vi "Test Command RPIN Response.vi"(8 "error in (no error)":errorcluster, 11 "TestCase in":refnum<class "Test ADC Command.lvclass">) -> (0 "error out":errorcluster, 3 "TestCase out":refnum<class "Test ADC Command.lvclass">)   [LabVIEW 2019, in "Test ADC Command.lvclass"]
uses:
  Test ADC Command.lvclass
  SIMULATED/SIMULATED.lvclass
  <vilib>/addons/_JKI Toolkits/VI Tester/TestCase.llb/TestCase.lvclass
  Serial Devices.lvclass
  C:/Program Files (x86)/National Instruments/LabVIEW 2019/vi.lib/addons/_JKI Toolkits/VI Tester/TestCase.llb/TestCase.lvclass
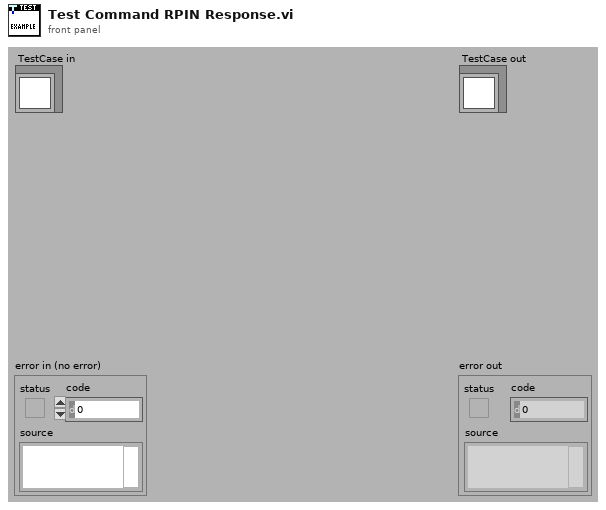
[diagram p1: front panel]
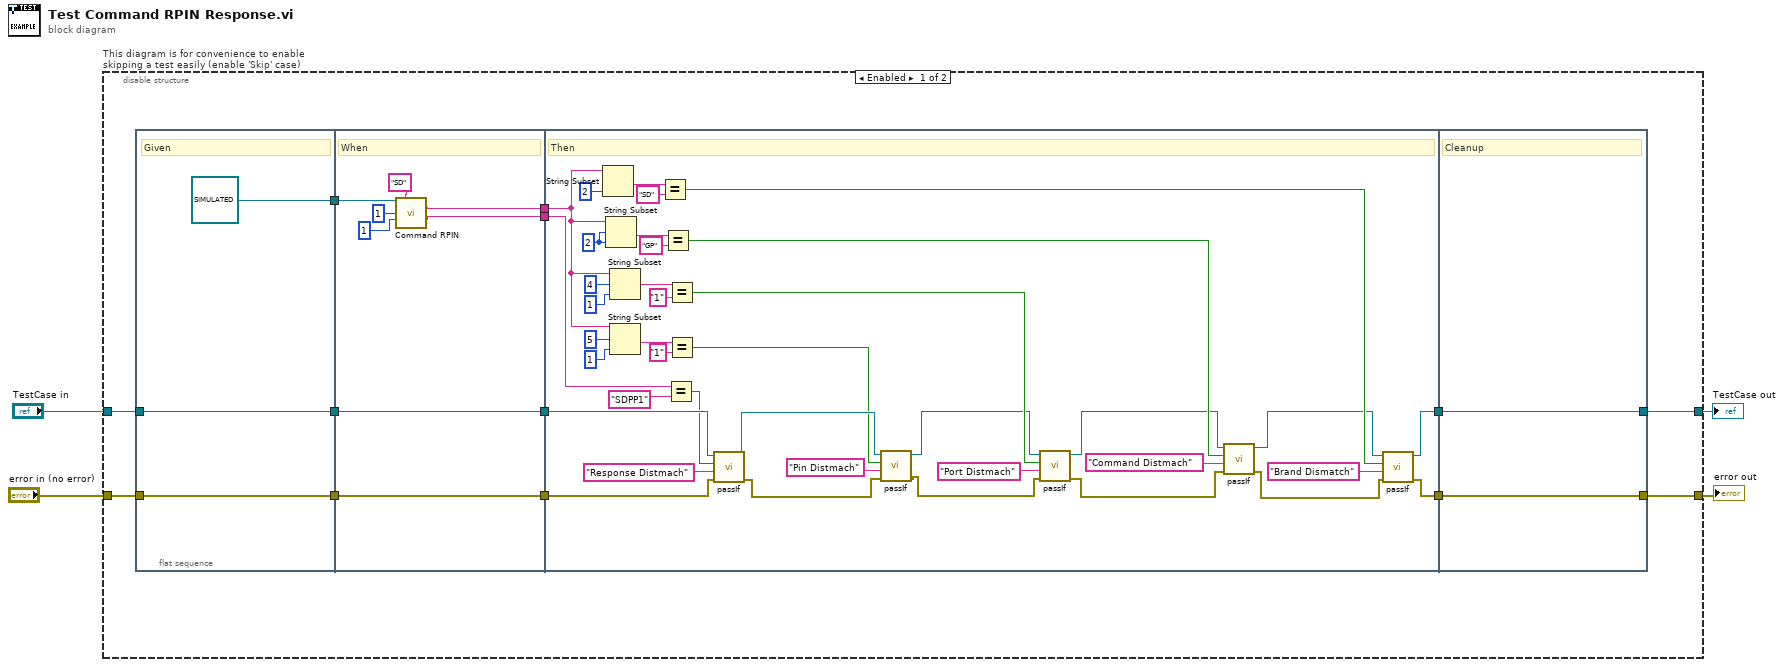
[diagram p0: block diagram]
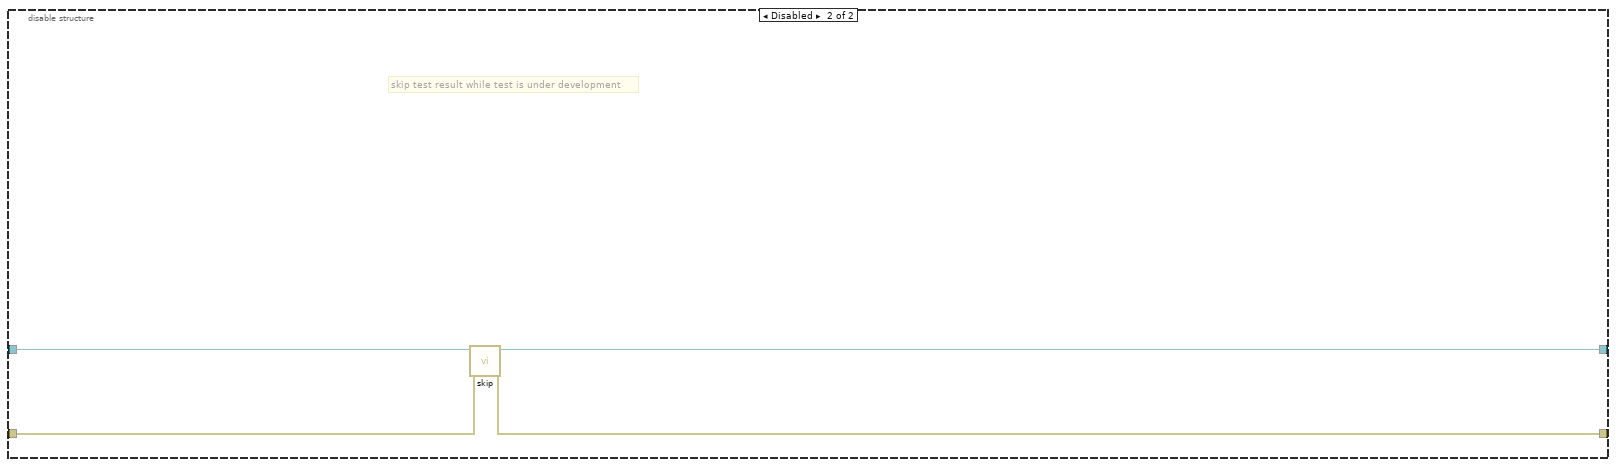
[diagram p2: hidden frame]
diagram:
  n1 = disable-structure "This diagram is for convenience to enable skipping a test easily (enable 'Skip' case)" shown="Enabled" {
    disable-tunnel: "TestCase in" -> [w16 w73]
    disable-tunnel: [w9 w71] -> w3
    disable-tunnel: [w8 w72] -> w4
    disable-tunnel: "error in (no error)" -> [w13 w70]
    frame Enabled {
      n2 = flat-sequence {
        tunnel: [w20] -> w17
        tunnel: w16 -> [w20]
        tunnel: [w19] -> w14
        tunnel: w13 -> [w19]
        tunnel: [refnum<class "SIMULATED.lvclass"> refnum ("SIMULATED.lvclass")] -> w7
        tunnel: w17 -> [w27]
        tunnel: [w27] -> w15
        tunnel: w14 -> [w28]
        tunnel: [w28] -> w12
        tunnel: w7 -> [w26]
        tunnel: [w25] -> w6
        tunnel: [w24] -> w5
        tunnel: w15 -> [w43]
        tunnel: w12 -> [w42]
        tunnel: [w62] -> w11
        tunnel: [w63] -> w10
        tunnel: w6 -> [w35]
        tunnel: w5 -> [w46]
        tunnel: [w69] -> w9
        tunnel: w11 -> [w69]
        tunnel: [w68] -> w8
        tunnel: w10 -> [w68]
        frame #0 {
          # "Given"
        }
        frame #1 {
          # "When"
          n3 = call "Command RPIN.vi"("Serial Devices in"=w26, "Device"="SD", "Port"=u8 1 ("Chanel"), "Pin"=u8 1 ("Chanel")) -> ("Command"=w25:string, "Expected"=w24:string)  [unwired: 8 in, 2 out]
        }
        frame #2 {
          w58 = 2 ("offset (0)")
          # "Then"
          n4 = String Subset(string=w35, length (rest)=2 ("offset (0)")) -> (substring=w66:string)  [unwired: 1 in]
          n5 = String Subset(string=w35, offset (0)=w58, length (rest)=w58) -> (substring=w59:string)
          n6 = String Subset(string=w35, offset (0)=4, length (rest)=1 ("length (rest)")) -> (substring=w36:string)
          n7 = String Subset(string=w35, offset (0)=5, length (rest)=1 ("length (rest)")) -> (substring=w38:string)
          n8 = Equal?(x=w66, y="SD") -> (x = y?=w64:bool)
          n9 = Equal?(x=w59, y="GP") -> (x = y?=w56:bool)
          n10 = Equal?(x=w46, y="SDPP1") -> (x = y?=w41:bool)
          n11 = Equal?(x=w36, y="1") -> (x = y?=w47:bool)
          n12 = Equal?(x=w38, y="1") -> (x = y?=w29:bool)
          n13 = call-dynamic "passIf.vi"("error in (no error)"=w42, "message (\"\")"="Response Distmach" ("message (\"\")"), "pass"=w41, "TestCase in"=w43) -> ("error out"=w30:errorcluster, "TestCase out"=w33:refnum<class "Test ADC Command.lvclass">)  [unwired: 6 in]
          n14 = call-dynamic "passIf.vi"("error in (no error)"=w30, "message (\"\")"="Pin Distmach" ("message (\"\")"), "pass"=w29, "TestCase in"=w33) -> ("error out"=w31:errorcluster, "TestCase out"=w32:refnum<class "Test ADC Command.lvclass">)  [unwired: 6 in]
          n15 = call-dynamic "passIf.vi"("error in (no error)"=w31, "message (\"\")"="Port Distmach" ("message (\"\")"), "pass"=w47, "TestCase in"=w32) -> ("error out"=w52:errorcluster, "TestCase out"=w54:refnum<class "Test ADC Command.lvclass">)  [unwired: 6 in]
          n16 = call-dynamic "passIf.vi"("error in (no error)"=w52, "message (\"\")"="Command Distmach" ("message (\"\")"), "pass"=w56, "TestCase in"=w54) -> ("error out"=w51:errorcluster, "TestCase out"=w57:refnum<class "Test ADC Command.lvclass">)  [unwired: 6 in]
          n17 = call-dynamic "passIf.vi"("error in (no error)"=w51, "message (\"\")"="Brand Dismatch" ("message (\"\")"), "pass"=w64, "TestCase in"=w57) -> ("error out"=w63:errorcluster, "TestCase out"=w62:refnum<class "Test ADC Command.lvclass">)  [unwired: 6 in]
        }
        frame #3 {
          # "Cleanup"
        }
      }
    }
    frame Disabled {
      # "skip test result while test is under development"
      n18 = call <vilib>:"skip.vi"("error in (no error)"=w70, "TestCase in"=w73) -> ("error out"=w72:errorcluster, "TestCase out"=w71:refnum<class "Test ADC Command.lvclass">)  [unwired: 8 in]
    }
  }
  "error out" <- w4
  "TestCase out" <- w3
